vi "__34401A_read_volt.vi"(7 "GPIB":string="22") -> (3 "Read_volt(mV)":dbl)   [LabVIEW 2017]
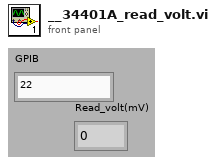
[diagram p1: front panel]
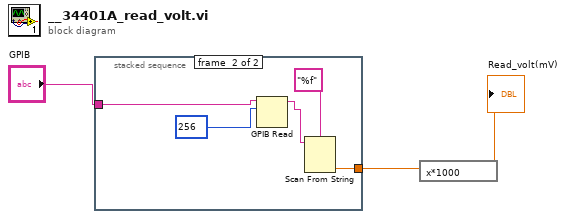
[diagram p0: block diagram]
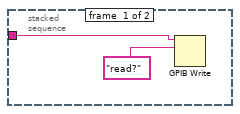
[diagram p2: hidden frame]
diagram:
  n1 = stacked-sequence {
    tunnel: "GPIB" -> [w5 w10]
    tunnel: [_ w6] -> w2
    frame #0 {
      n2 = GPIB Write(0:w5, 1:"read?") -> ()  [unwired: 3 in, 2 out]
    }
    frame #1 {
      n3 = GPIB Read(0:w10, 1:256) -> (5:w7:string)  [unwired: 3 in, 2 out]
      n4 = Scan From String(format string="%f", input string=w7) -> (output 1=w6:dbl)  [unwired: 3 in, 3 out]
    }
  }
  n5 = expression code="x*1000"(w2) -> (→"Read_volt(mV)":dbl)
